vi "Get Module Main Status.vi"(8 "error in":errorcluster, 10 "Library in":refnum<vi>, 11 "application Instance":refnum<vi>) -> (0 "error out":errorcluster, 1 "Module Exec State":T1(ring), 2 "Library Name":string)   [LabVIEW 2020, in "Panther Dashboard.lvlib"]
uses:
  Panther Dashboard.lvlib
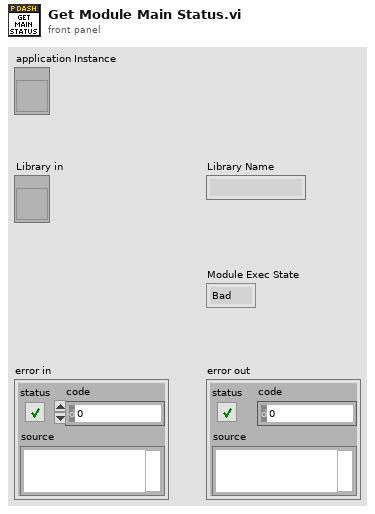
[diagram p1: front panel]
types:
  T1 = enum32{"Bad", "Idle", "Run top level", "Running"}
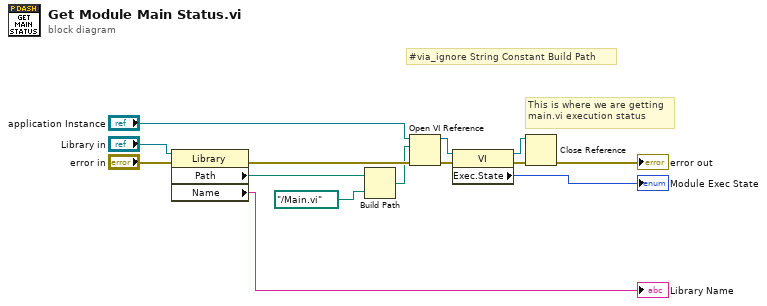
[diagram p0: block diagram]
diagram:
  # "#via_ignore String Constant Build Path"
  # "This is where we are getting\nmain.vi execution status"
  n1 = property class="Library"(reference="Library in", error in="error in") -> (error out=w10:errorcluster, "Path"=w5:path, "Name"=→"Library Name":string)  [unwired: 1 out]
  n2 = Build Path(base path=w5, name or relative path=path "../Main.vi") -> (appended path=w6:path)
  n3 = Open VI Reference(application reference (local)="application Instance", vi path=w6, error in (no error)=w10) -> (vi reference=w7:refnum<vi>, error out=w14:errorcluster)  [unwired: 3 in]
  n4 = property class="VI"(reference=w7, error in=w14) -> (reference out=w8:refnum<vi>, error out=w13:errorcluster, "Exec.State"=→"Module Exec State":T1)
  n5 = Close Reference(reference=w8, error in (no error)=w13) -> (error out=→"error out":errorcluster)
